vi "mask_rpc.vi"() -> ()   [LabVIEW 2017]
panel:
  in  "address":string="192.168.10.35"
  out "Array 3":u8[][](array[numeric])=[[0, 1, 2, 3, 4, 5, 6, 7], [136, 137, 138, 139, 140, 141, 142, 143], [16, 17, 18, 19, 20, 21, 22, 23], [24, 25, 26, 27, 28, 29, 30, 31], [32, 33, 34, 35, 36, 37, 38, 39], [40, 41, 42, 43, 44, 45, 46, 47], [48, 49, 50, 51, 52, 53, 54, 55], [56, 57, 58, 59, 60, 61, 62, 63], [64, 65, 66, 67, 68, 69, 70, 71], [72, 73, 74, 75, 76, 77, 78, 79]] format="%x"
  in  "Array 2":bool[][](array[boolean])=[[FALSE, FALSE, FALSE, FALSE, FALSE, FALSE, FALSE, FALSE], [FALSE, FALSE, FALSE, FALSE, FALSE, FALSE, FALSE, FALSE], [FALSE, FALSE, FALSE, FALSE, FALSE, FALSE, FALSE, FALSE], [FALSE, FALSE, FALSE, FALSE, FALSE, FALSE, FALSE, FALSE], [FALSE, FALSE, FALSE, FALSE, FALSE, FALSE, FALSE, FALSE], [FALSE, FALSE, FALSE, FALSE, FALSE, FALSE, FALSE, FALSE], [FALSE, FALSE, FALSE, FALSE, FALSE, FALSE, FALSE, FALSE], [FALSE, FALSE, FALSE, FALSE, FALSE, FALSE, FALSE, FALSE], [FALSE, FALSE, FALSE, FALSE, FALSE, FALSE, FALSE, FALSE], [FALSE, FALSE, FALSE, FALSE, FALSE, FALSE, FALSE, FALSE]]
  in  "error in (no error)":errorcluster
  out "error out":errorcluster
  out "In 2":u8=79 format="%.0x"
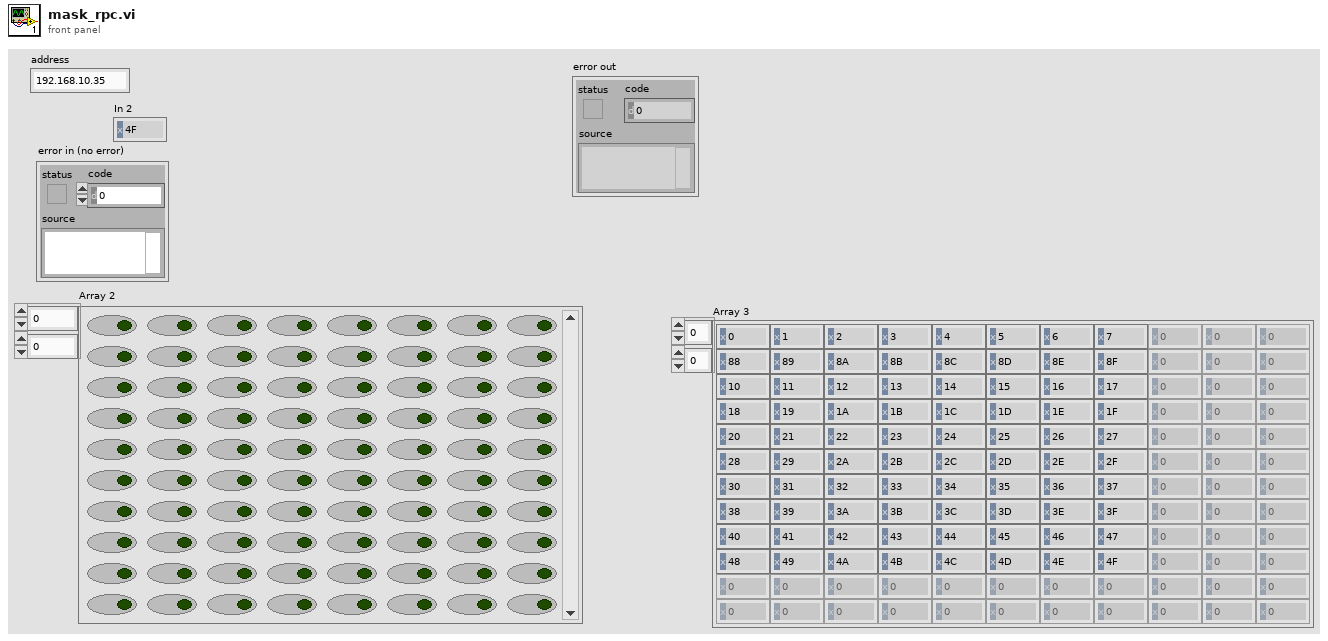
[diagram p1: front panel]
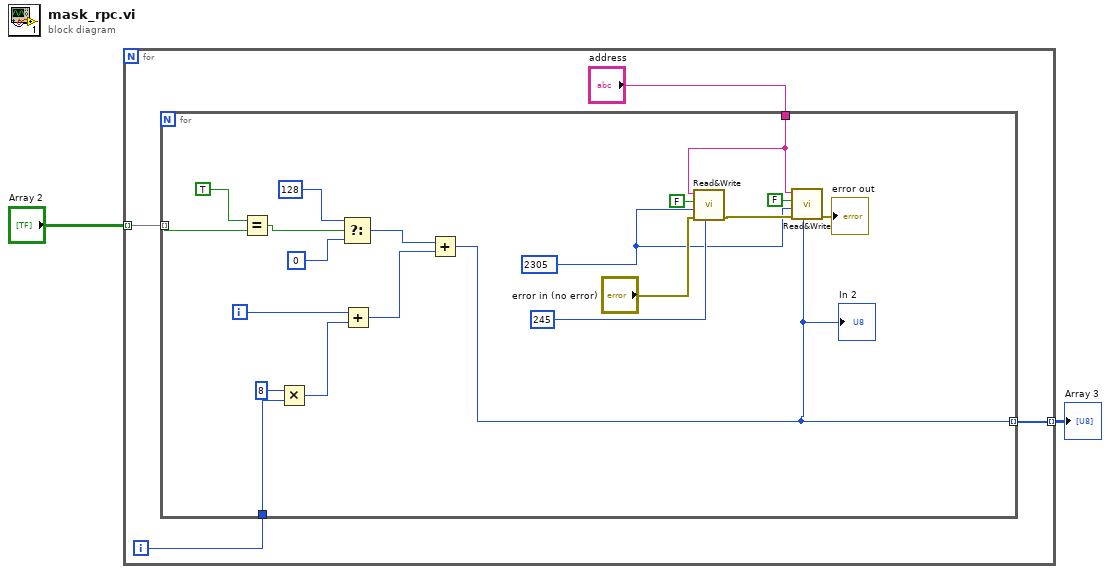
[diagram p0: block diagram]
diagram:
  n1 = for {
    tunnel: "Array 2" -> [w5] mode=indexing
    tunnel: [w3] -> w1 mode=indexing
    i -> [w4]
    n2 = for {
      tunnel: w5 -> [w19] mode=indexing
      tunnel: "address" -> [w20]
      tunnel: w4 -> [w13]
      tunnel: [w8] -> w3 mode=indexing
      i -> [w10]
      w7 = u32 2305 ("Address")
      n3 = Equal?(x=TRUE, y=w19) -> (x = y?=w17:bool)
      n4 = Multiply(x=8, y=w13) -> (x*y=w11:i32)
      n5 = Select(t=u8 128 ("In 3"), s=w17, f=u8 0 ("In 3")) -> (s? t:f=w15:u8)
      n6 = Add(x=w10, y=w11) -> (x+y=w9:i32)
      n7 = Add(x=w15, y=w9) -> (x+y=w8:i32)
      "In 2" <- w8
      n8 = call "Read&Write.vi"("In"=u8 245, "error in (no error)"="error in (no error)", "Address"=w7, "Read (TRUE)"=FALSE, "address"=w20) -> ("error out"=w26:errorcluster)  [unwired: 5 in, 1 out]
      n9 = call "Read&Write.vi"("In"=w8, "error in (no error)"=w26, "Address"=w7, "Read (TRUE)"=FALSE, "address"=w20) -> ("error out"=→"error out":errorcluster)  [unwired: 5 in, 1 out]
    }
  }
  "Array 3" <- w1
